vi "Modify accounts.vi"(8 "error in":errorcluster, 9 "Users data":T1, 10 "User input":string, 11 "Account action":T4) -> (0 "error out":errorcluster, 1 "Message":T3, 2 "User input output":string, 3 "Users data out":T1)   [LabVIEW 2015]
doc: "Validate password.\nAdd maney to account.\nWithdraw money from account."
uses:
  Controls/Account action.ctl
  Controls/Users data.ctl
  Controls/user.ctl
  Controls/Message.ctl
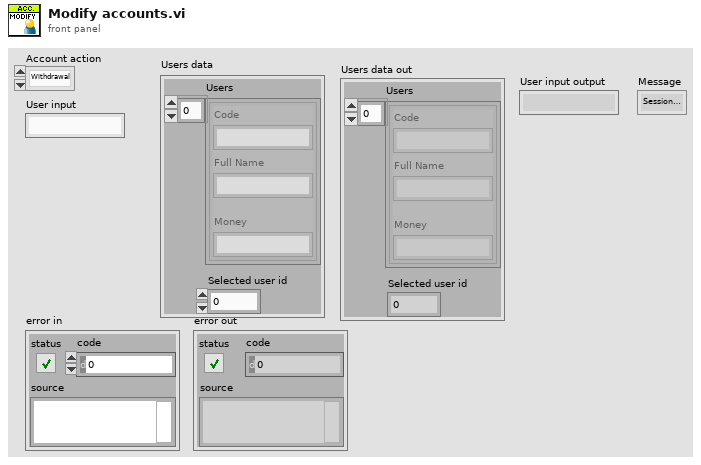
[diagram p1: front panel]
types:
  T1 = typedef "Users data.ctl" = cluster{"Users":T2[], "Selected user id":i32}
  T2 = typedef "user.ctl" = cluster{"Code":string, "Full Name":string, "Money":string}
  T3 = typedef "Message.ctl" = enum16{"Session Terminate ", "Account Verification Failed", "Main Menu ", "Balance Inquiry", "Withdrawal Failed", "Withdrawal Complete", "Withdrawal", "Deposit Complete", "Deposit ", "Welcome "}
  T4 = typedef "Account action.ctl" = enum16{"Withdrawal", "Balance", "Deposit", "Validation"}
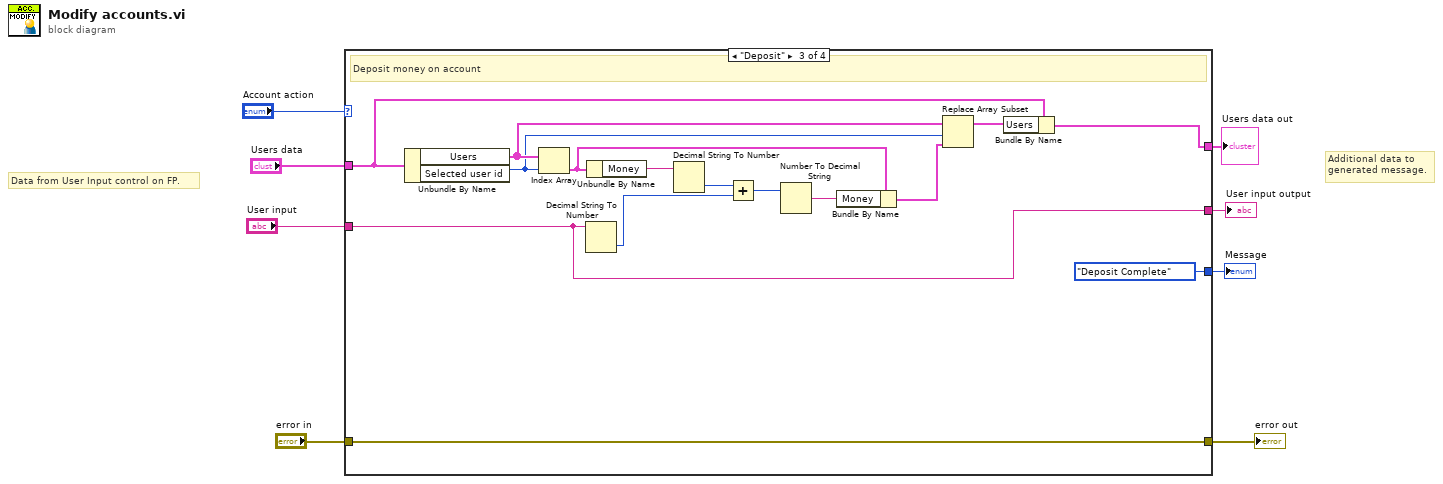
[diagram p0: block diagram]
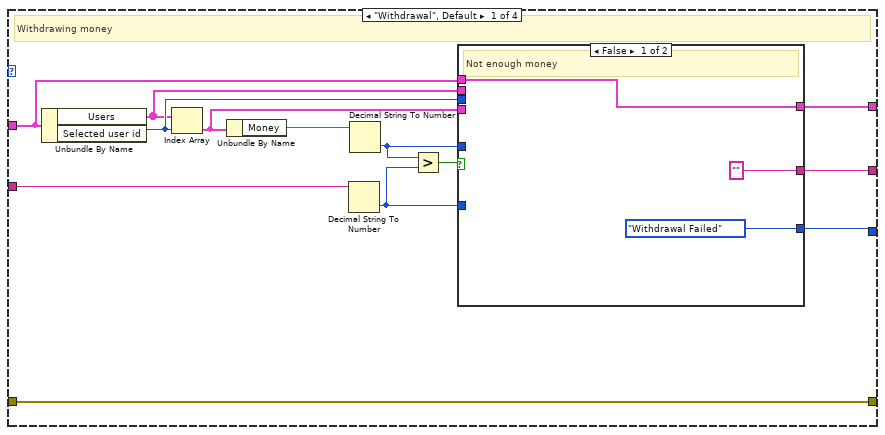
[diagram p2: hidden frame]
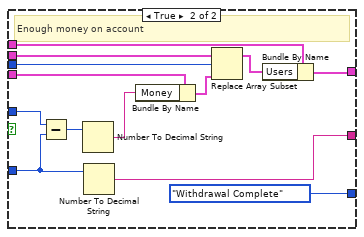
[diagram p3: hidden frame]
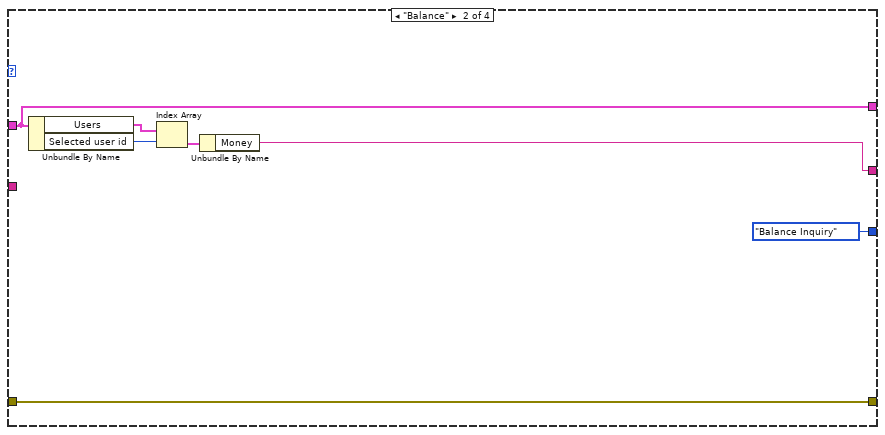
[diagram p4: hidden frame]
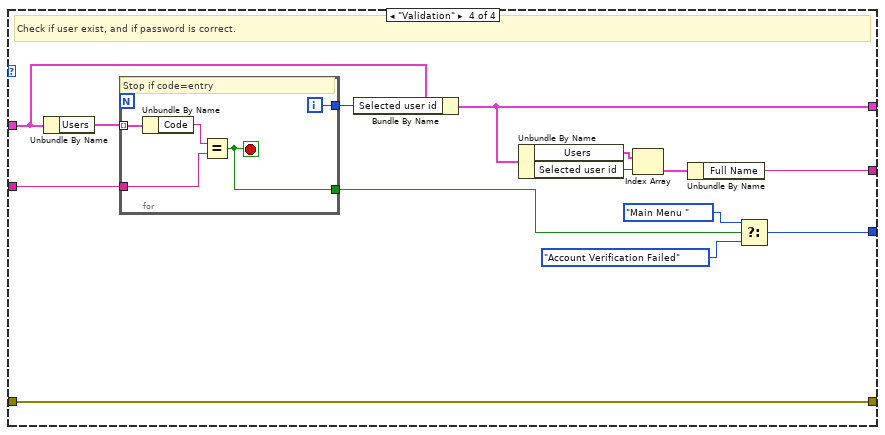
[diagram p5: hidden frame]
diagram:
  # "Additional data to\ngenerated message."
  # "Data from User Input control on FP."
  n1 = case shown="\"Deposit\"" "Account action" {
    tunnel: "Users data" -> [w16 w40 w50 w70]
    tunnel: "User input" -> [w20 _ w57 w72]
    tunnel: [w9 w38 w47 w73] -> w6
    tunnel: "error in" -> [w9 w38 w47 w73]
    tunnel: [w15 w40 w48 w68] -> w3
    tunnel: [w17 w41 w57 w64] -> w2
    tunnel: [w18 Message."Balance Inquiry" ("Message") Message."Deposit Complete" ("Message") w60] -> w1
    frame "Withdrawal", Default {
      # "Withdrawing money"
      n2 = Unbundle By Name(w16) -> ("Users"=w10:T2[], "Selected user id"=w11:i32)
      n3 = Index Array(array=w10, index=w11) -> (element=w12:T2)
      n4 = Unbundle By Name(w12) -> ("Money"=w21:string)
      n5 = Decimal String To Number(string=w20) -> (number=w13:i32)  [unwired: 2 in, 1 out]
      n6 = Decimal String To Number(string=w21) -> (number=w14:i32)  [unwired: 2 in, 1 out]
      n7 = Greater?(x=w14, y=w13) -> (0:w19:bool)
      n8 = case shown="False" w19 {
        tunnel: [Message."Withdrawal Failed" ("Message") Message."Withdrawal Complete" ("Message")] -> w18
        tunnel: ["" w33] -> w17
        tunnel: w16 -> [w22 w30]
        tunnel: [w22 w25] -> w15
        tunnel: w14 -> [_ w36]
        tunnel: w13 -> [_ w34]
        tunnel: w12 -> [_ w32]
        tunnel: w11 -> [_ w28]
        tunnel: w10 -> [_ w29]
        frame False {
          # "Not enough money"
        }
        frame True {
          # "Enough money on account"
          n9 = Subtract(x=w36, y=w34) -> (x-y=w35:i32)
          n10 = Number To Decimal String(number=w35) -> (decimal integer string=w31:string)  [unwired: 1 in]
          n11 = Number To Decimal String(number=w34) -> (decimal integer string=w33:string)  [unwired: 1 in]
          n12 = Bundle By Name(cluster=w32, "Money"=w31) -> (w27:T2)
          n13 = Replace Array Subset(array=w29, new element=w27, index=w28) -> (w26:T2[])
          n14 = Bundle By Name(cluster=w30, "Users"=w26) -> (w25:T1)
        }
      }
    }
    frame "Balance" {
      n15 = Unbundle By Name(w40) -> ("Users"=w44:T2[], "Selected user id"=w43:i32)
      n16 = Index Array(array=w44, index=w43) -> (element=w42:T2)
      n17 = Unbundle By Name(w42) -> ("Money"=w41:string)
    }
    frame "Deposit" {
      # "Deposit money on account"
      n18 = Unbundle By Name(w50) -> ("Users"=w53:T2[], "Selected user id"=w52:i32)
      n19 = Index Array(array=w53, index=w52) -> (element=w55:T2)
      n20 = Decimal String To Number(string=w57) -> (number=w45:i32)  [unwired: 2 in, 1 out]
      n21 = Unbundle By Name(w55) -> ("Money"=w59:string)
      n22 = Decimal String To Number(string=w59) -> (number=w58:i32)  [unwired: 2 in, 1 out]
      n23 = Add(x=w58, y=w45) -> (x+y=w56:i32)
      n24 = Number To Decimal String(number=w56) -> (decimal integer string=w54:string)  [unwired: 1 in]
      n25 = Bundle By Name(cluster=w55, "Money"=w54) -> (w51:T2)
      n26 = Replace Array Subset(array=w53, new element=w51, index=w52) -> (w49:T2[])
      n27 = Bundle By Name(cluster=w50, "Users"=w49) -> (w48:T1)
    }
    frame "Validation" {
      # "Check if user exist, and if password is correct."
      n28 = Unbundle By Name(w70) -> ("Users"=w71:T2[])
      n29 = for {
        tunnel: w71 -> [w78] mode=indexing
        tunnel: w72 -> [w76]
        tunnel: [w75] -> w69
        tunnel: [w74] -> w63
        i -> [w75]
        stop <- w74 stop-if-true
        # "Stop if code=entry"
        n30 = Unbundle By Name(w78) -> ("Code"=w77:string)
        n31 = Equal?(x=w77, y=w76) -> (x = y?=w74:bool)
      }
      n32 = Bundle By Name(cluster=w70, "Selected user id"=w69) -> (w68:T1)
      n33 = Unbundle By Name(w68) -> ("Users"=w66:T2[], "Selected user id"=w67:i32)
      n34 = Index Array(array=w66, index=w67) -> (element=w65:T2)
      n35 = Unbundle By Name(w65) -> ("Full Name"=w64:string)
      n36 = Select(t=Message."Main Menu " ("Message"), s=w63, f=Message."Account Verification Failed" ("Message")) -> (s? t:f=w60:T3)
    }
  }
  "error out" <- w6
  "Users data out" <- w3
  "User input output" <- w2
  "Message" <- w1
